vi "readREFfilter.vi"(5 "Port":u16, 7 "address":string, 8 "error in (no error)":errorcluster, 11 "Instrument.Lockin in":refnum<class "Instrument.Lockin.lvclass">) -> (0 "error out":errorcluster, 2 "REF filter":T1={"TC (s)"=0.3, "order"=2} {"TC (s)" format="%#_6p"}, 3 "Instrument.Lockin out":refnum<class "Instrument.Lockin.lvclass">)   [LabVIEW 2016]
doc: "API to get the results of lockin calculation.\n\nIf address=\"\", this API reads from localhost\nIf address is remote lockin, you need to add this computer to allowed whitelist on the lockin computer you are trying to access."
uses:
  Instrument.Lockin/Typedefs/REF filter-cluster.ctl
  Instrument.Lockin/Instrument.Lockin.lvclass
  Instrument.Lockin/Typedefs/Instrument.Lockin.Commands--Enum.ctl
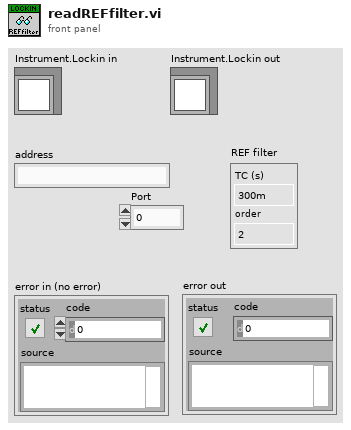
[diagram p1: front panel]
types:
  T1 = typedef "Instrument.Lockin.lvclass/REF filter-cluster.ctl" = cluster{"TC (s)":dbl, "order":i32}
  T2 = typedef "Instrument.Lockin.lvclass/Instrument.Lockin.Commands--Enum.ctl" = enum16{"configAO", "configAO_Amplitude", "configAO_DC", "configAO_Frequency", "configAO_Phase", "configAO_Function", "configAO_I+", "configREF", "configREF_Frequency", "configREF_Phase", "configREF_Filter", "configIVmode", "Reset", "configSampling", "Trigger", "getAO", "getAI", "getResults", "getTrigger", "getIVmode", "getSampling", "getAOconfig", "getREFconfig", "getREF_Filter", "configGain", "getGain"}
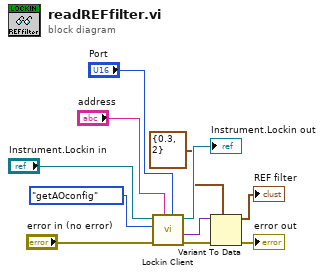
[diagram p0: block diagram]
diagram:
  n1 = call "Lockin Client.vi"("Port"="Port", "address"="address", "error in (no error)"="error in (no error)", "Command"=Instrument.Lockin.Commands--Enum."getAOconfig", "Instrument.Lockin in"="Instrument.Lockin in") -> ("error out"=w8:errorcluster, "Data out"=w9:variant, "Instrument.Lockin out"=→"Instrument.Lockin out":refnum<class "Instrument.Lockin.lvclass">)  [unwired: 4 in]
  n2 = Variant To Data(error in=w8, type=T1 {"TC (s)"=0.3, "order"=2} ("REF filter"), Variant=w9) -> (data=→"REF filter":T1, error out=→"error out":errorcluster)
